vi "Actor Core.vi"(8 "error in":errorcluster, 11 "User Interface in":refnum<class "User Interface.lvclass">) -> (0 "error out":errorcluster, 3 "Actor out":refnum<class "Actor.lvclass">)   [LabVIEW 2015, in "User Interface.lvlib" / "User Interface.lvclass"]
doc: "(<B>Filename</B>: Actor Framework.lvlib:Actor.lvclass:Actor Core.vi)\n\nReceives messages to the actor, reacts to them, and initiates any error handling that may shut the actor down.\n\nDescendant classes may override this VI to append parallel tasks for the actor to complete while it handles messages. Overrides use the Call Parent Method node."
uses:
  User Interface.lvclass
  <vilib>/ActorFramework/Actor/Actor.lvclass
  Controls/Car Position.ctl
  Controls/Wash Entry.ctl
  Controls/Car Wash Indicators.ctl
  Controls/Wash Options.ctl
  <vilib>/ActorFramework/Actor/Actor.lvclass/Actor.ctl
  <vilib>/ActorFramework/Message Enqueuer/Message Enqueuer.lvclass/Message Enqueuer.ctl
  User Interface.lvclass/User Interface.ctl
  Controller/Controller Messages/Ask Wash Parameters Msg/Ask Wash Parameters Msg.lvclass/Ask Wash Parameters Msg.ctl
  <vilib>/ActorFramework/Message Enqueuer/Init from Existing Queue.vi
  <vilib>/ActorFramework/Message Enqueuer/Enqueue.vi
  <vilib>/ActorFramework/Message Priority Queue/Priority Enqueue.vi
  <vilib>/ActorFramework/Message Enqueuer/Message Enqueuer.lvclass
  <vilib>/ActorFramework/Stop Msg/Stop Msg.lvclass
  Controller/Controller Messages/Ask Wash Parameters Msg/Ask Wash Parameters Msg.lvclass
panel:
  out "Elapsed Time":dbl format="%#.2f"
  in  "Start":bool
  in  "Wash Options":T1
  out "Car Wash Indicators":T2
  out "Wash Entry":T3
  out "Car Position Slider":T4 max=2 scale=0.0..2.0
  in  "Stop":bool
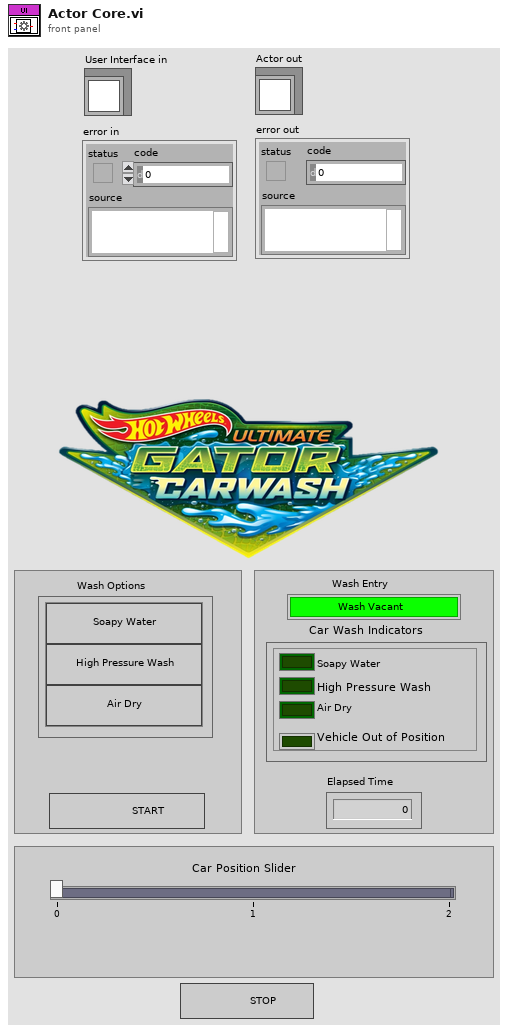
[diagram p1: front panel]
types:
  T1 = typedef "Wash Options.ctl" = cluster{"Soapy Water":bool, "High Pressure Wash":bool, "Air Dry":bool}
  T2 = typedef "Car Wash Indicators.ctl" = cluster{"Soapy Water":bool, "High Pressure Wash":bool, "Air Dry":bool, "Vehicle Out of Position":bool}
  T3 = typedef "Wash Entry.ctl" = bool
  T4 = typedef "Car Position.ctl" = u8
  T5 = enum32{"Invalid", "Standard", "Closed", "Hidden", "Minimized", "Maximized"}
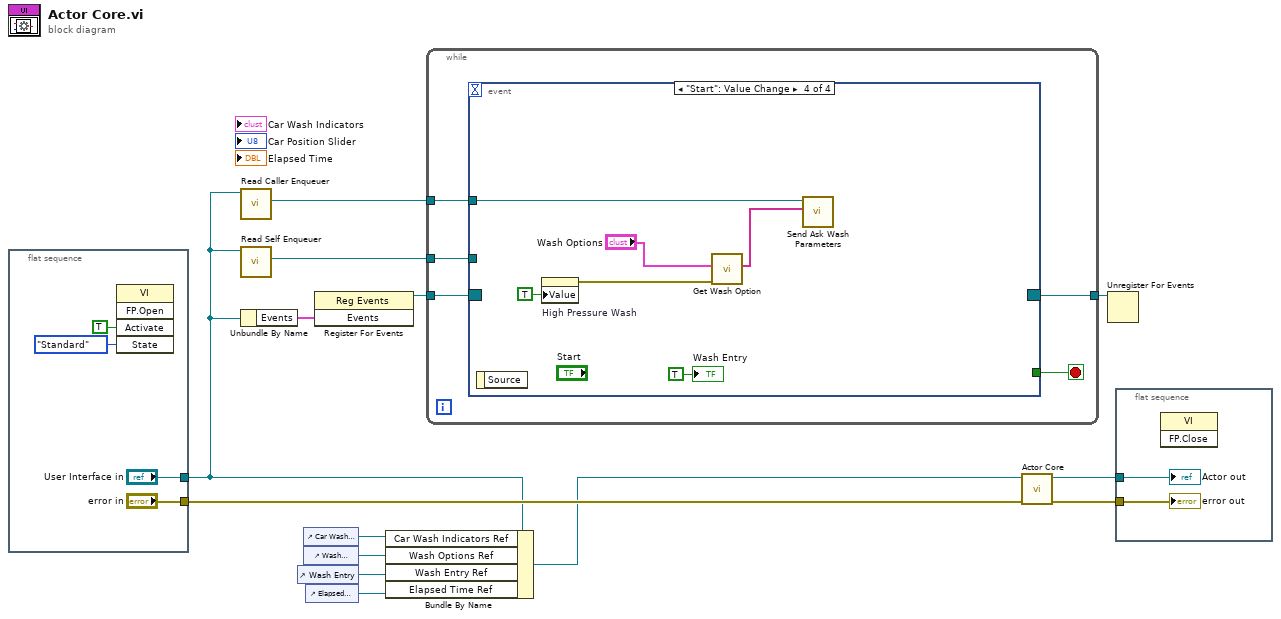
[diagram p0: block diagram]
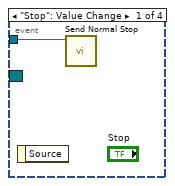
[diagram p2: hidden frame]
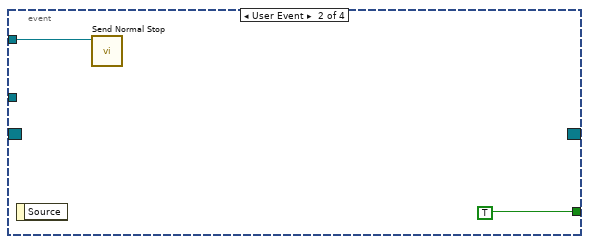
[diagram p3: hidden frame]
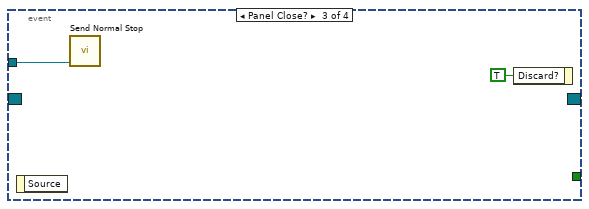
[diagram p4: hidden frame]
diagram:
  n1 = flat-sequence {
    tunnel: ["error in"] -> w12
    tunnel: ["User Interface in"] -> w8
    frame #0 {
      n2 = invoke class="VI" method="FP.Open"("Activate"=TRUE ("Activate?"), "State"=T5."Standard") -> ()  [unwired: 3 in, 5 out]
    }
  }
  n3 = call <vilib>:"Read Caller Enqueuer.vi"("Actor"=w8) -> ("Caller Enqueuer"=w11:refnum<class "Message Enqueuer.lvclass">)  [unwired: 10 in]
  n4 = call <vilib>:"Read Self Enqueuer.vi"("Actor"=w8) -> ("Self Enqueuer"=w10:refnum<class "Message Enqueuer.lvclass">)  [unwired: 10 in]
  n5 = Unbundle By Name(w8) -> ("Events"=w7:cluster{"Stop event":refnum<user-event>})
  n6 = control-ref of="Wash Entry"() -> (w2:refnum<vi>)
  n7 = control-ref of="Car Wash Indicators"() -> (w4:refnum<vi>)
  n8 = control-ref of="Wash Options"() -> (w3:refnum<vi>)
  n9 = control-ref of="Elapsed Time"() -> (w1:refnum<vi>)
  n10 = register-events(w7) -> (reference out=w6:refnum<event-registration>)  [unwired: 2 in, 1 out]
  n11 = Bundle By Name(cluster=w8, "Car Wash Indicators Ref"=w4, "Wash Options Ref"=w3, "Wash Entry Ref"=w2, "Elapsed Time Ref"=w1) -> (w5:refnum<class "User Interface.lvclass">)
  n12 = while {
    tunnel: w11 -> [w23]
    tunnel: w10 -> [w22]
    tunnel: [w21] -> w9
    tunnel: w6 -> [w20]
    stop <- w19 stop-if-true
    n13 = event shown="[3] \"Start\": Value Change" {
      selector: w20 -> [_ _ _ _]
      dyn-events: [_ _ _ _] -> w21
      timeout: _ -> [_ _ _ _]
      tunnel: w22 -> [w24 _ w27 _]
      tunnel: w23 -> [_ w25 _ w30]
      tunnel: [_ TRUE _ _] -> w19
      event "Stop": Value Change {
        n14 = event-data() -> ()  [unwired: 1 in, 1 out]
        n15 = call <vilib>:"Send Normal Stop.vi"("Message Enqueuer"=w24) -> ()  [unwired: 10 in, 1 out]
      }
      event User Event {
        n16 = event-data() -> ()  [unwired: 1 in, 1 out]
        n17 = call <vilib>:"Send Normal Stop.vi"("Message Enqueuer"=w25) -> ()  [unwired: 10 in, 1 out]
      }
      event Panel Close? {
        n18 = event-data() -> ()  [unwired: 1 in, 1 out]
        n19 = call <vilib>:"Send Normal Stop.vi"("Message Enqueuer"=w27) -> ()  [unwired: 10 in, 1 out]
        n20 = event-data("Discard?"=TRUE) -> ()  [unwired: 1 in, 1 out]
      }
      event "Start": Value Change {
        n21 = event-data() -> ()  [unwired: 1 in, 1 out]
        n22 = property on="High Pressure Wash" class="Bool (strict)"("Value"=TRUE) -> (error out=w31:errorcluster)  [unwired: 2 in, 1 out]
        n23 = call "Get Wash Option.vi"("Error In"=w31, "Wash Options"="Wash Options") -> ("Option Name"=w29:string[])  [unwired: 8 in, 1 out]
        n24 = call "Send Ask Wash Parameters.vi"("Car Option"=w29, "Message Enqueuer"=w30) -> ()  [unwired: 8 in, 2 out]
        "Wash Entry" <- T3 TRUE ("Wash Entry")
      }
    }
  }
  n25 = call-parent "Actor Core.vi"("error in"=w12, "Actor in"=w5) -> ("error out"=w14:errorcluster, "Actor out"=w13:refnum<class "Actor.lvclass">)  [unwired: 8 in]
  n26 = Unregister For Events(event registration refnum=w9) -> ()  [unwired: 1 in, 1 out]
  n27 = flat-sequence {
    tunnel: w14 -> [w36]
    tunnel: w13 -> [w35]
    frame #0 {
      n28 = invoke class="VI" method="FP.Close"() -> ()  [unwired: 3 in, 3 out]
      "error out" <- w36
      "Actor out" <- w35
    }
  }
